vi "PSCUI_Temp Variable.vi"() -> (2 "TmpData":T2)   [LabVIEW 2016]
uses:
  X-Analysis/SubVIs/VCH/Private/Ctrls/PSVCH_All Channels.ctl
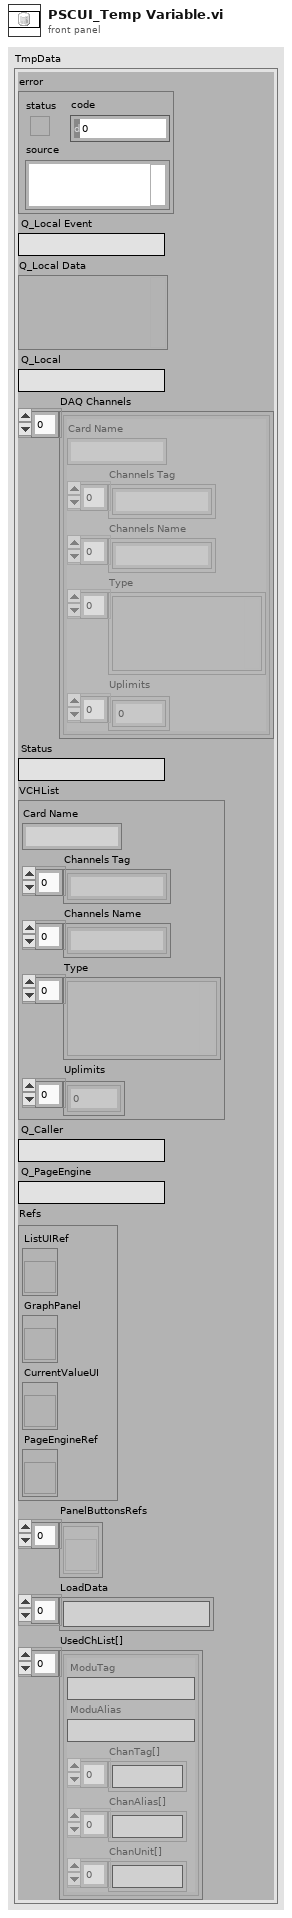
[diagram p1: front panel]
types:
  T1 = typedef "PSVCH_All Channels.ctl" = cluster{"Card Name":string, "Channels Tag":string[], "Channels Name":string[], "Type":variant[], "Uplimits":dbl[]}
  T2 = cluster{"error":errorcluster, "Q_Local Event":string, "Q_Local Data":variant, "Q_Local":string, "DAQ Channels":T1[], "Status":string, "VCHList":T1, "Q_Caller":string, "Q_PageEngine":string, "Refs":cluster{"ListUIRef":refnum<vi>, "GraphPanel":refnum<vi>, "CurrentValueUI":refnum<vi>, "PageEngineRef":refnum<vi>}, "PanelButtonsRefs":refnum<vi>[], "LoadData":string[], "UsedChList[]":cluster{"ModuTag":string, "ModuAlias":string, "ChanTag[]":string[], "ChanAlias[]":string[], "ChanUnit[]":string[]}[]}
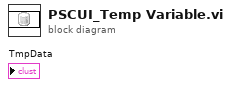
[diagram p0: block diagram]
diagram:
